vi "Do Core.vi"(8 "error in (no error)":errorcluster, 9 "Actor in":refnum<class "Actor.lvclass">, 11 "Divide Msg.lvclass":refnum<class "Divide Msg.lvclass">) -> (0 "error out":errorcluster, 1 "Actor out":refnum<class "Actor.lvclass">, 2 "Variant":variant)   [LabVIEW 2020, in "Messaging Tests.lvlib" / "Divide Msg.lvclass"]
uses:
  Divide Msg.lvclass
  Divide Msg.lvclass/Divide Msg.ctl
  Increment Msg/Increment Msg.lvclass
  C:/dev/actor-framework/dist/vi.lib/ActorFramework/Message/Message.lvclass
  C:/dev/actor-framework/dist/Test/Unit Tests/Core/Messaging Tests/TestActor/Increment Msg/Increment Msg.lvclass
  Test Actor/TestActor.lvclass
  C:/dev/actor-framework/dist/vi.lib/ActorFramework/Actor/Actor.lvclass
  C:/dev/actor-framework/dist/Test/Unit Tests/Core/Messaging Tests/TestActor/Test Actor/TestActor.lvclass
  vi.lib/ActorFramework/Actor/Actor.lvclass
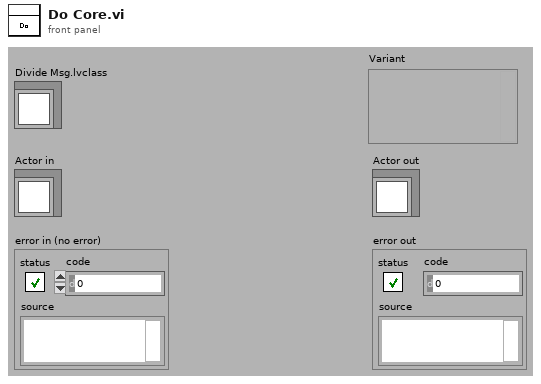
[diagram p1: front panel]
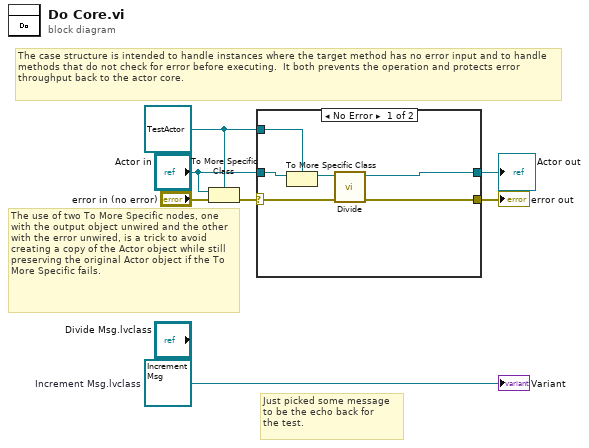
[diagram p0: block diagram]
diagram:
  w1 = refnum<class "Increment Msg.lvclass"> refnum  # Increment Msg.lvclass
  w4 = refnum<class "TestActor.lvclass"> refnum ("Actor in")
  # "Just picked some message\nto be the echo back for\nthe test."
  # "The use of two To More Specific nodes, one with the output object unwired and the other with the error unwired, is a trick to avoid creating a copy of the Actor object while still preserving the original Actor object if the To More Specific fails."
  # "The case structure is intended to handle instances where the target method has no error input and to handle methods that do not check for error before executing.  It both prevents the operation and protects error throughput back to the actor core."
  n1 = To More Specific Class(target class=w4, reference="Actor in", error in="error in (no error)") -> (error out=w7:errorcluster)  [unwired: 1 out]
  n2 = case shown="No Error" w7 {
    selector: w7 -> [w12 w15]
    tunnel: [w13 w15] -> w5
    tunnel: [w11 w14] -> w2
    tunnel: "Actor in" -> [w10 w14]
    tunnel: w4 -> [w9 _]
    frame No Error {
      n3 = To More Specific Class(target class=w9, reference=w10) -> (specific class reference=w8:refnum<class "TestActor.lvclass">)  [unwired: 1 in, 1 out]
      n4 = call "Divide.vi"("error in (no error)"=w12, "TestActor in"=w8) -> ("error out"=w13:errorcluster, "TestActor out"=w11:refnum<class "TestActor.lvclass">)  [unwired: 8 in]
    }
    frame Error {
      # "If type check fails, pass the original object out again."
    }
  }
  "Actor out" <- w2
  "error out" <- w5
  "Variant" <- w1
